vi "Keyence.Cmd.Read.vi"(8 "error in (no error)":errorcluster, 9 "Timeout [ms] (1000)":i32=1000, 10 "Bank":u8, 11 "connection ID":refnum<k5>) -> (0 "error out":errorcluster, 1 "read ok":bool, 2 "Code":T1, 3 "connection ID out":refnum<k5>)   [LabVIEW 2016]
uses:
  Keyence.CodeDetails.ctl
panel:
  out "command":string
  out "code string":string
  out "response":string
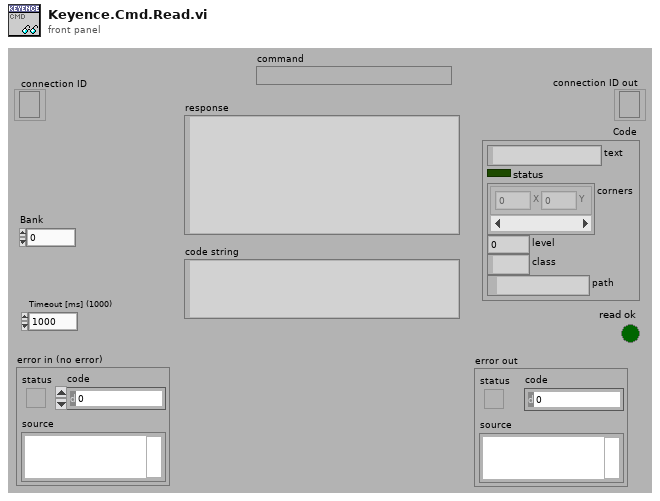
[diagram p1: front panel]
types:
  T1 = typedef "Keyence.CodeDetails.ctl" = cluster{"text":string, "status":bool, "corners":cluster{"X":i32, "Y":i32}[], "level":u8, "class":string, "path":path}
  T2 = enum16{"Standard", "Buffered", "CRLF", "Immediate"}
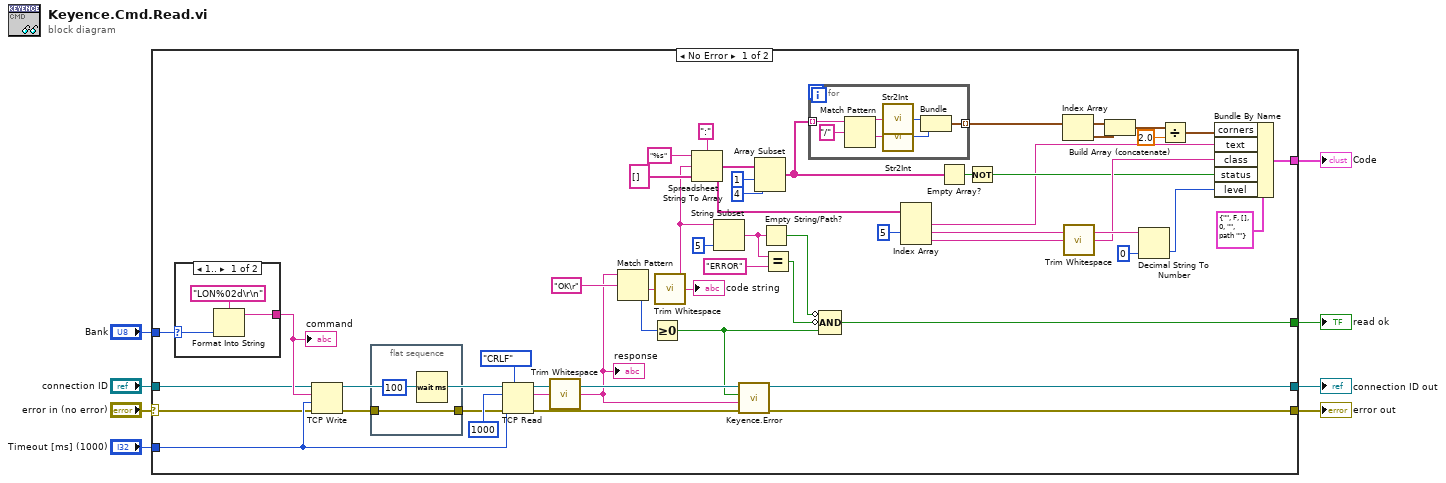
[diagram p0: block diagram]
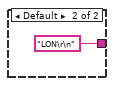
[diagram p2: hidden frame]
diagram:
  n1 = case shown="No Error" "error in (no error)" {
    selector: "error in (no error)" -> [w40 w72]
    tunnel: [w37 w72] -> w8
    tunnel: "Timeout [ms] (1000)" -> [w57 _]
    tunnel: [w10 _] -> w5
    tunnel: "connection ID" -> [w42 w71]
    tunnel: "Bank" -> [w41 _]
    tunnel: [w39 w71] -> w2
    tunnel: [w20 _] -> w1
    frame No Error {
      n2 = case shown="1.." w41 {
        selector: w41 -> [w67 _]
        tunnel: [w66 "LON\r\n" ("concatenated string")] -> w51
        frame 1.. {
          n3 = Format Into String(format string="LON%02d\r\n" ("concatenated string"), w67) -> (resulting string=w66:string)  [unwired: 2 in, 1 out]
        }
        frame Default {
        }
      }
      "command" <- w51
      n4 = TCP Write(connection ID=w42, data in=w51, error in (no error)=w40, 9:w57) -> (connection ID out=w56:refnum<k5>, error out=w53:errorcluster)  [unwired: 1 out]
      n5 = flat-sequence {
        tunnel: w53 -> [w70]
        tunnel: [w70] -> w52
        frame #0 {
          n6 = Wait (ms)(milliseconds to wait=u32 100) -> ()  [unwired: 1 out]
        }
      }
      n7 = TCP Read(connection ID=w56, bytes to read=1000, error in (no error)=w52, 7:T2."CRLF" ("mode (standard)"), 9:w57) -> (connection ID out=w39:refnum<k5>, data out=w49:string, error out=w50:errorcluster)
      n8 = call <vilib>:"Trim Whitespace.vi"("string"=w49) -> ("trimmed string"=w35:string)  [unwired: 1 in]
      "response" <- w35
      n9 = Match Pattern(string=w35, regular expression="OK\r") -> (after substring=w46:string, offset past match=w47:i32)  [unwired: 1 in, 2 out]
      n10 = Greater Or Equal To 0?(x=w47) -> (x >= 0?=w36:bool)
      n11 = call <vilib>:"Trim Whitespace.vi"("string"=w46) -> ("trimmed string"=w22:string)  [unwired: 1 in]
      "code string" <- w22
      n12 = Spreadsheet String To Array(delimiter (Tab)=":" ("regular expression"), format string="%s", spreadsheet string=w22, array type (2D Dbl)=string[] []) -> (array=w13:string[])
      n13 = String Subset(string=w22, length (rest)=5 ("length (rest)")) -> (substring=w43:string)  [unwired: 1 in]
      n14 = call "Keyence.Error.vi"("error in (no error)"=w50, "Response"=w35, "Cmd ok"=w36) -> ("error out"=w37:errorcluster)  [unwired: 8 in]
      n15 = Array Subset(array=w13, index=1, length=4 ("index")) -> (w16:string[])
      n16 = Empty String/Path?(string/path=w43) -> (empty?=w38:bool)
      n17 = Equal?(x=w43, y="ERROR") -> (x = y?=w11:bool)
      n18 = for {
        tunnel: w16 -> [w61] mode=indexing
        tunnel: [w58] -> w31 mode=indexing
        n19 = Match Pattern(string=w61, regular expression="/") -> (before substring=w63:string, after substring=w62:string)  [unwired: 1 in, 2 out]
        n20 = call "Str2Int.vi"("string"=w63) -> ("Numeric"=w60:i32)
        n21 = call "Str2Int.vi"("string"=w62) -> ("Numeric"=w59:i32)
        n22 = Bundle("Numeric"=w60, "Numeric"=w59) -> (w58:cluster{"Numeric":i32, "Numeric":i32})  [unwired: 1 in]
      }
      n23 = Compound Arithmetic op=AND(invert w38, invert w11, w36) -> (w10:bool)
      n24 = Index Array(array=w13, index #2=5 ("index")) -> (element #1=w9:string, element #2=w23:string, element #3=w24:string)  [unwired: 2 in]
      n25 = Empty Array?(array=w16) -> (empty?=w15:bool)
      n26 = Not(x=w15) -> (.not. x?=w12:bool)
      n27 = Index Array(array=w31) -> (element=w30:cluster{"Numeric":i32, "Numeric":i32})  [unwired: 1 in]
      n28 = call <vilib>:"Trim Whitespace.vi"("string"=w24) -> ("trimmed string"=w18:string)  [unwired: 1 in]
      n29 = Build Array (concatenate)(w31, w30) -> (w28:cluster{"Numeric":i32, "Numeric":i32}[])
      n30 = Decimal String To Number(string=w23, default (0L)=u8 0 ("default (0 I32)")) -> (number=w17:u8)  [unwired: 2 out]
      n31 = Divide(x=w28, y=2.0) -> (x/y=w27:cluster{"Numeric":dbl, "Numeric":dbl}[])
      n32 = Bundle By Name(cluster=T1 {"text"="", "status"=FALSE, "corners"=[], "level"=0, "class"="", "path"=path ""} ("Code details"), "corners"=w27, "text"=w9, "class"=w18, "status"=w12, "level"=w17) -> (w20:T1)
    }
    frame Error {
    }
  }
  "error out" <- w8
  "read ok" <- w5
  "connection ID out" <- w2
  "Code" <- w1
